vi "Joystick 1 Button Handler.vi"(8 "error in (no error)":errorcluster, 11 "Buttons":bool[](array[boolean])) -> (0 "error out":errorcluster)   [LabVIEW 2015]
uses:
  <vilib>/Rock Robotics/WPI/Solenoid/WPI_SolenoidValue.ctl
  <vilib>/Rock Robotics/WPI/Solenoid/WPI_SolenoidSetEnum.vi
  <vilib>/Rock Robotics/WPI/Solenoid/WPI_SolenoidGetEnum.vi
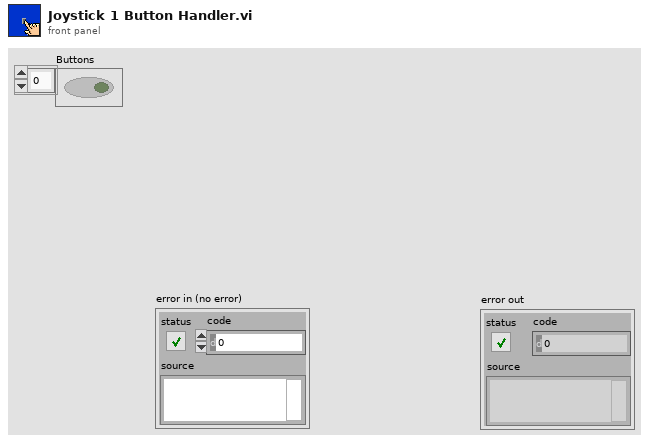
[diagram p1: front panel]
types:
  T1 = typedef "WPI_SolenoidValue.ctl" = enum16{"Off", "On", "Forward", "Reverse"}
  T2 = typedef "WPI_SolenoidDevRef.ctl" = cluster{"DevStatus":errorcluster, "Pneumatics Control Module":u8, "Forward Solenoid Channel":T3, "Reverse Solenoid Channel":T3}
  T3 = typedef "WPI_SolenoidChannel.ctl" = enum8{"Solenoid 0", "Solenoid 1", "Solenoid 2", "Solenoid 3", "Solenoid 4", "Solenoid 5", "Solenoid 6", "Solenoid 7", "Invalid"}
  T4 = typedef "WPI_MotorControlDeviceRef.ctl" = cluster{"DeviceStatus":errorcluster, "Type":T5, "PWM":cluster{"PWM Channel":T6, "DeadBand":T7}, "CAN":cluster{"Device Number":u8, "Control Mode":T8, "Semaphore":T9, "Max Vout":dbl, "TalonSRX Control Mode":T10}, "Invert":bool}
  T5 = typedef "WPI_MotorControlType.ctl" = enum16{"PWM", "CAN", "CANTalonSRX"}
  T6 = typedef "FPGA_DIOPWMChannel.ctl" = enum8{"PWM 0", "PWM 1", "PWM 2", "PWM 3", "PWM 4", "PWM 5", "PWM 6", "PWM 7", "PWM 8", "PWM 9", "PWM MXP 0", "PWM MXP 1", "PWM MXP 2", "PWM MXP 3", "PWM MXP 4", "PWM MXP 5", "PWM MXP 6", "PWM MXP 7", "PWM MXP 8", "PWM MXP 9", "Invalid"}
  T7 = typedef "WPI_PWMDeadband.ctl" = cluster{"Name":string, "maxPositivePwm":i32, "minPositivePwm":i32, "centerPwm":i32, "maxNegativePwm":i32, "minNegativePwm":i32, "angularRange":u16}
  T8 = typedef "WPI_CANJaguar_ControlMode.ctl" = enum8{"Percent VBus", "Current", "Speed", "Position", "Voltage"}
  T9 = typedef "Semaphore RefNum" = refnum<k1>
  T10 = typedef "WPI_CANTalonSRX_APIControlMode.ctl" = enum8{"Percent VBus", "Speed", "Position", "Slave", "Unchanged / Invalid", "Voltage Compensation", "Current", "Motion Profile"}
  T11 = typedef "WPI_DigitalInputDevRef.ctl" = cluster{"DevStatus":errorcluster, "DIO Channel":T12}
  T12 = typedef "FPGA_DIOChannel.ctl" = enum8{"DIO 0", "DIO 1", "DIO 2", "DIO 3", "DIO 4", "DIO 5", "DIO 6", "DIO 7", "DIO 8", "DIO 9", "DIO MXP 0", "DIO MXP 1", "DIO MXP 2", "DIO MXP 3", "DIO MXP 4", "DIO MXP 5", "DIO MXP 6", "DIO MXP 7", "DIO MXP 8", "DIO MXP 9", "DIO MXP 10", "DIO MXP 11", "DIO MXP 12", "DIO MXP 13", "DIO MXP 14", "DIO MXP 15", "Invalid"}
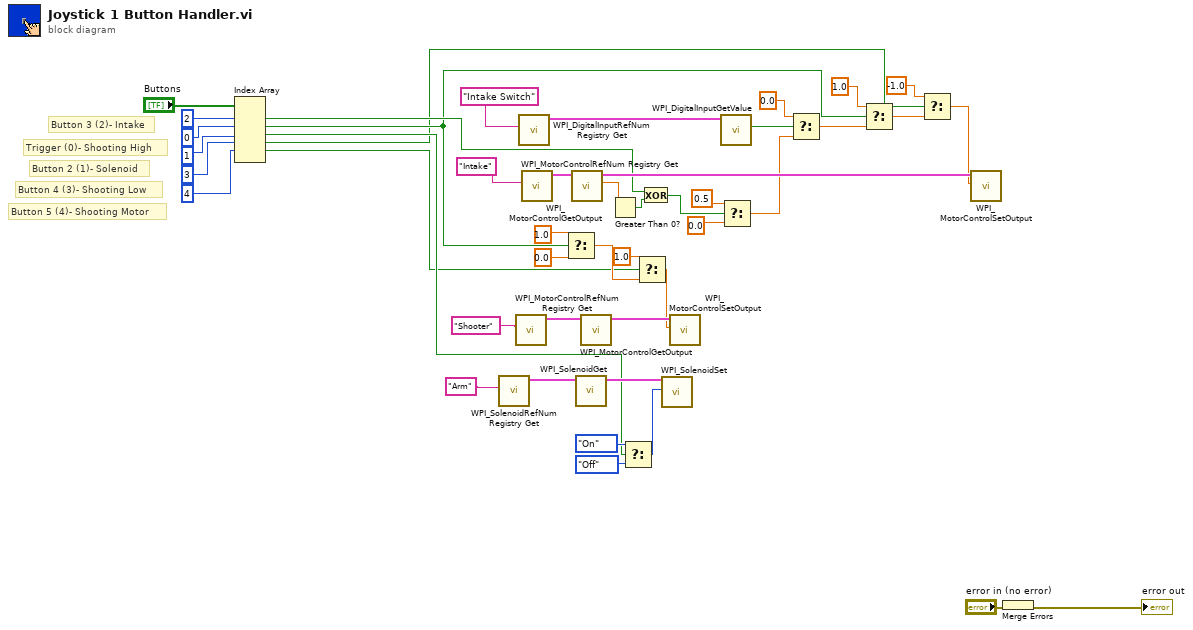
[diagram p0: block diagram]
diagram:
  # "Button 5 (4)- Shooting Motor"
  # "Button 4 (3)- Shooting Low"
  # "Button 2 (1)- Solenoid"
  # "Trigger (0)- Shooting High"
  # "Button 3 (2)- Intake"
  n1 = Index Array(array="Buttons", index #1=2 ("index"), index #2=0 ("index"), index #3=1 ("index"), index #4=3 ("index"), index #5=4 ("index")) -> (element #1=w31:bool, element #2=w27:bool, element #3=w12:bool, element #4=w9:bool, element #5=w1:bool)  [unwired: 1 in, 1 out]
  n2 = call <vilib>:"WPI_SolenoidRefNum Registry Get.vi"("refnum name"="Arm") -> ("SolenoidDevRef"=w17:T2)  [unwired: 9 in, 1 out]
  n3 = call <vilib>:"WPI_MotorControlRefNum Registry Get.vi"("refnum name"="Shooter") -> ("MotorControlDevRef"=w24:T4)  [unwired: 9 in, 1 out]
  n4 = call <vilib>:"WPI_DigitalInputRefNum Registry Get.vi"("refnum name"="Intake Switch") -> ("DigitalInputDevRef"=w40:T11)  [unwired: 9 in, 1 out]
  n5 = call <vilib>:"WPI_MotorControlRefNum Registry Get.vi"("refnum name"="Intake") -> ("MotorControlDevRef"=w38:T4)  [unwired: 9 in, 1 out]
  n6 = Select(t=1.0, s=w27, f=0.0) -> (s? t:f=w4:dbl)
  n7 = call <vilib>:"WPI_MotorControlGetOutput.vi"("MotorControlDevRef"=w38) -> ("Output"=w33:dbl, "MotorControlDevRef"=w37:T4)  [unwired: 8 in, 1 out]
  n8 = call-poly <vilib>:"WPI_SolenoidGet.vi"("SolenoidDevRef"=w17) -> ("SolenoidDevRef"=w15:T2)  [unwired: 8 in, 2 out]
  n9 = call <vilib>:"WPI_MotorControlGetOutput.vi"("MotorControlDevRef"=w24) -> ("MotorControlDevRef"=w26:T4)  [unwired: 8 in, 2 out]
  n10 = Greater Than 0?(x=w33) -> (x > 0?=w36:bool)
  n11 = Select(t=WPI_SolenoidValue."On" ("Value"), s=w12, f=WPI_SolenoidValue."Off" ("Value")) -> (s? t:f=w11:T1)
  n12 = Select(t=1.0, s=w1, f=w4) -> (s? t:f=w2:dbl)
  n13 = Exclusive Or(1:w36, 2:w31) -> (0:w19:bool)
  n14 = call-poly <vilib>:"WPI_SolenoidSet.vi"("Value"=w11, "SolenoidDevRef"=w15) -> ()  [unwired: 8 in, 2 out]
  n15 = call <vilib>:"WPI_MotorControlSetOutput.vi"("Output"=w2, "MotorControlDevRef"=w26) -> ()  [unwired: 7 in, 3 out]
  n16 = call <vilib>:"WPI_DigitalInputGetValue.vi"("DigitalInputDevRef"=w40) -> ("Value"=w35:bool)  [unwired: 8 in, 2 out]
  n17 = Select(t=0.5, s=w19, f=0.0) -> (s? t:f=w21:dbl)
  n18 = Select(t=0.0, s=w35, f=w21) -> (s? t:f=w20:dbl)
  n19 = Select(t=1.0, s=w27, f=w20) -> (s? t:f=w10:dbl)
  n20 = Select(t=-1.0, s=w9, f=w10) -> (s? t:f=w7:dbl)
  n21 = call <vilib>:"WPI_MotorControlSetOutput.vi"("Output"=w7, "MotorControlDevRef"=w37) -> ()  [unwired: 7 in, 3 out]
  n22 = Merge Errors("error in (no error)") -> (→"error out":errorcluster)
